vi "tect conflict.vi"() -> ()   [LabVIEW 2019]
uses:
  Stand_class/Valve Mode.ctl
  FPGA/TypeDef/DO index.ctl
  8e5458a2-6e96-40e0-bc2b-84d63334d380.vi
  67e4eee1-ce7f-4ac0-a553-d55e8c92af70.vi
  99c42b3a-ad8d-4631-9065-e98a8dfe7a8b.vi
  9a9bede7-f2be-4a12-8a6a-bc68bae3e033.vi
  196b6594-7a50-4d11-8096-5ae1f87b325d.vi
  5a27167f-4186-4e0b-ad76-77799e900baa.vi
  Stand_class/Valve State Mode.vi/810e184e-eeb6-4027-a8ae-1422f3ce3d45.vi
  Stand_class/Valve State Mode.vi/57bd4a65-f3dc-44f5-8d68-677c2a197570.vi
  Stand_class/Valve State Mode.vi/03b2f9e4-fceb-4725-9b90-3fd10082a088.vi
  Stand_class/Valve State Mode.vi/3d0d09bd-48e8-482f-b1e2-a36b2bb65234.vi
  Stand_class/Valve State Mode.vi/33d3f26a-dc4a-4f56-bf0a-61d04c5d7434.vi
  Stand_class/Valve State Mode.vi/52af9d47-24d1-4057-80bf-8d93bfb3d17d.vi
  Stand_class/Valve State Mode.vi/094228cb-a119-423c-9af8-5a16f059a318.vi
  Stand_class/Valve State Mode.vi/bf5ad1e6-a0ae-4579-ad74-ca8f304cb7cf.vi
  Stand_class/Valve State Mode.vi/eb4d2b76-f0f0-4e1d-bda0-609c5f37b4e7.vi
  Stand_class/Const All Valve.vi
panel:
  out "OK":bool
  out "intersection 2":set{T1}(c389)
  out "intersection 1":set{T1}(c389)
  in  "Valve Mode 2":T2
  in  "Valve Mode 1":T2
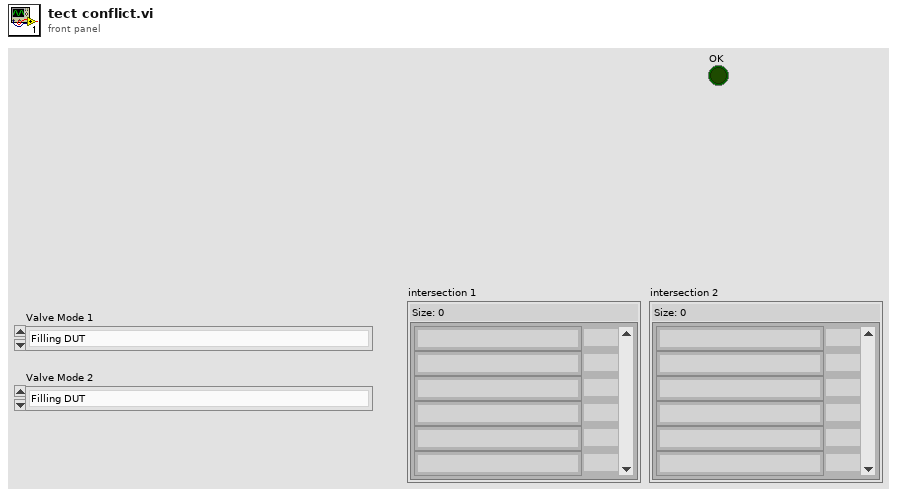
[diagram p1: front panel]
types:
  T1 = typedef "DO index.ctl" = u8
  T2 = typedef "Valve Mode.ctl" = enum16{"Filling DUT", "Filling Chamber", "Pump Pressure DUT", "Pump Pressure Chamber", "Haskel Pressure DUT", "Haskel Pressure Chamber", "Slow Release DUT", "Slow Release Chamber", "Fast Release DUT", "Fast Release Chamber", "Fast Release DUT and Chamber", "Leak Pressure DUT", "Leak Pressure Chamber", "Back Pressure DUT", "Back Pressure Chamber", "Fully Closed"}
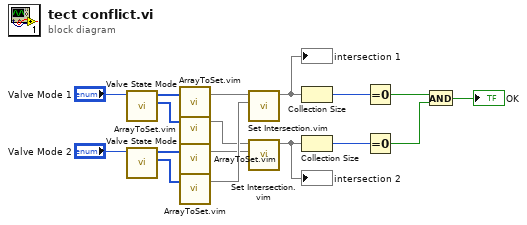
[diagram p0: block diagram]
diagram:
  n1 = call "Valve State Mode.vi"("Valve Mode"="Valve Mode 1") -> ("close"=w9:T1[], "open"=w14:T1[])  [unwired: 9 in]
  n2 = call "Valve State Mode.vi"("Valve Mode"="Valve Mode 2") -> ("close"=w15:T1[], "open"=w8:T1[])  [unwired: 9 in]
  n3 = call "ArrayToSet.vim"("Array"=w14) -> ("Set"=w13:set{T1})  [unwired: 2 in]
  n4 = call "ArrayToSet.vim"("Array"=w9) -> ("Set"=w10:set{T1})  [unwired: 2 in]
  n5 = call "ArrayToSet.vim"("Array"=w8) -> ("Set"=w11:set{T1})  [unwired: 2 in]
  n6 = call "ArrayToSet.vim"("Array"=w15) -> ("Set"=w12:set{T1})  [unwired: 2 in]
  n7 = call "Set Intersection.vim"("set 2"=w12, "set 1"=w13) -> ("intersection"=w7:set{T1})  [unwired: 9 in]
  "intersection 1" <- w7
  n8 = call "Set Intersection.vim"("set 2"=w11, "set 1"=w10) -> ("intersection"=w6:set{T1})  [unwired: 9 in]
  "intersection 2" <- w6
  n9 = Collection Size(1:w7) -> (0:w4:i32)
  n10 = Collection Size(1:w6) -> (0:w5:i32)
  n11 = Equal To 0?(x=w4) -> (x = 0?=w3:bool)
  n12 = Equal To 0?(x=w5) -> (x = 0?=w2:bool)
  n13 = And(x=w3, y=w2) -> (x .and. y?=→"OK":bool)
